vi "reset.vi"(8 "error in (no error)":errorcluster, 11 "PsuNiPxi in":refnum<class "PsuNi.lvclass">) -> (0 "error out":errorcluster, 3 "PsuNiPxi out":refnum<class "PsuNi.lvclass">)   [LabVIEW 2023, in "PsuNi.lvclass"]
doc: "<b>Author:</b> Wolfgang\n<b>Description:</b> This method is used to reset the instrument to a default and known state."
uses:
  PsuNi.lvclass
  PsuNi.lvclass/PsuNi.ctl
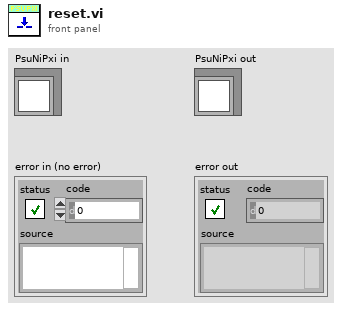
[diagram p1: front panel]
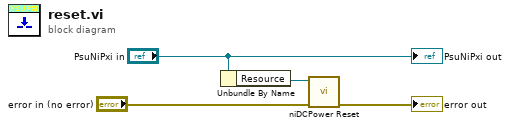
[diagram p0: block diagram]
diagram:
  n1 = Unbundle By Name("PsuNiPxi in") -> ("Resource"=w3:refnum<k15>)
  n2 = call <instrlib>:"niDCPower Reset.vi"("error in (no error)"="error in (no error)", "instrument handle"=w3) -> ("error out"=→"error out":errorcluster)  [unwired: 8 in, 1 out]
  "PsuNiPxi out" <- "PsuNiPxi in"
